vi "Choose Retical.vi"(10 "Image In":T2, 11 "Climb Retical":bool) -> (3 "Image Out":T2)   [LabVIEW 2012]
uses:
  <vilib>/vision/Image Controls.llb/IMAQ Image.ctl
panel:
  in  "Rectangle":T1={"Left"=125, "Top"=133, "Right"=195, "Bottom"=152}
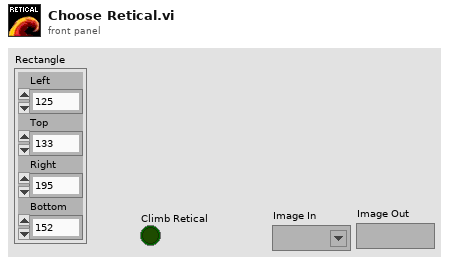
[diagram p1: front panel]
types:
  T1 = cluster{"Left":i32, "Top":i32, "Right":i32, "Bottom":i32}
  T2 = typedef "IMAQ Image.ctl" = refnum<image>
  T3 = enum16{"Shooting Rect", "Pin Shooting", "Climbing"}
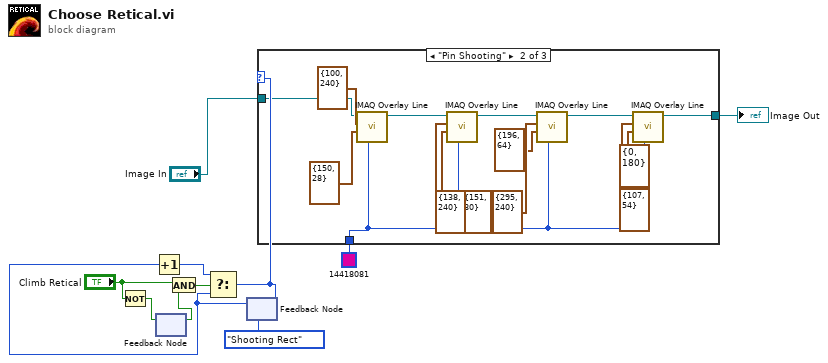
[diagram p0: block diagram]
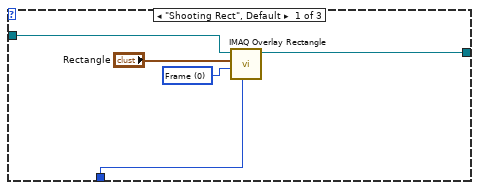
[diagram p2: hidden frame]
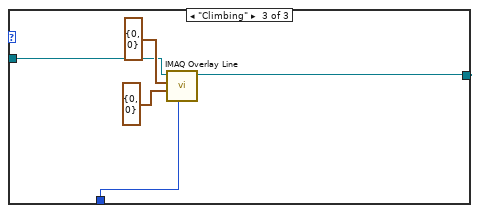
[diagram p3: hidden frame]
diagram:
  n1 = Not(x="Climb Retical") -> (.not. x?=w7:bool)
  n2 = feedback #1() -> (w8:bool)  [unwired: 1 in]
  n3 = feedback-in #1(w7) -> ()
  n4 = And(x="Climb Retical", y=w8) -> (x .and. y?=w6:bool)
  n5 = feedback #2(T3."Shooting Rect" ("Enum")) -> (w4:T3)
  n6 = Increment(x=w4) -> (x+1=w5:T3)
  n7 = Select(t=w5, s=w6, f=w4) -> (s? t:f=w2:T3)
  n8 = feedback-in #2(w2) -> ()
  n9 = case shown="\"Pin Shooting\"" w2 {
    tunnel: "Image In" -> [w15 w26 w33]
    tunnel: [w14 w18 w32] -> w10
    tunnel: u32 14418081 ("Color") -> [w13 w17 w31]
    frame "Shooting Rect", Default {
      w12 = u32 0 items=["Frame", "Fill", "Highlight"] ("Drawing Mode (Frame)")
      n10 = call "IMAQ Overlay Rectangle"("Color"=w13, "Drawing Mode (Frame)"=w12, "Rectangle"="Rectangle", "Image"=w15) -> ("Image Out"=w14:T2)  [unwired: 6 in, 1 out]
    }
    frame "Pin Shooting" {
      n11 = call "IMAQ Overlay Line"("Color"=w17, "End Point"=cluster{"X":i32, "Y":i32} {"X"=150, "Y"=28} ("Start Point"), "Start Point"=cluster{"X":i32, "Y":i32} {"X"=100, "Y"=240} ("End Point"), "Image"=w26) -> ("Image Out"=w28:T2)  [unwired: 6 in, 1 out]
      n12 = call "IMAQ Overlay Line"("Color"=w17, "End Point"=cluster{"X":i32, "Y":i32} {"X"=151, "Y"=80} ("Start Point 2"), "Start Point"=cluster{"X":i32, "Y":i32} {"X"=138, "Y"=240} ("End Point 2"), "Image"=w28) -> ("Image Out"=w27:T2)  [unwired: 6 in, 1 out]
      n13 = call "IMAQ Overlay Line"("Color"=w17, "End Point"=cluster{"X":i32, "Y":i32} {"X"=196, "Y"=64} ("Start Point 3"), "Start Point"=cluster{"X":i32, "Y":i32} {"X"=295, "Y"=240} ("End Point 3"), "Image"=w27) -> ("Image Out"=w19:T2)  [unwired: 6 in, 1 out]
      n14 = call "IMAQ Overlay Line"("Color"=w17, "End Point"=cluster{"X":i32, "Y":i32} {"X"=107, "Y"=54} ("Start Point 4"), "Start Point"=cluster{"X":i32, "Y":i32} {"X"=0, "Y"=180} ("End Point 4"), "Image"=w19) -> ("Image Out"=w18:T2)  [unwired: 6 in, 1 out]
    }
    frame "Climbing" {
      n15 = call "IMAQ Overlay Line"("Color"=w31, "End Point"=cluster{"X":i32, "Y":i32} {"X"=0, "Y"=0} ("Climb Begin"), "Start Point"=cluster{"X":i32, "Y":i32} {"X"=0, "Y"=0} ("Climb End"), "Image"=w33) -> ("Image Out"=w32:T2)  [unwired: 6 in, 1 out]
    }
  }
  "Image Out" <- w10
